vi "Initialize.vi"(8 "error in (no error)":errorcluster) -> (0 "error out":errorcluster, 3 "LiDAR out":refnum<class "Telnet V2.lvclass">)   [LabVIEW 2018]
uses:
  Telnet V2.lvclass
  PPLs/Configuration/Configuration.lvlibp/Configuration.lvclass
  C:/AME Test Engineering/LabVIEW/PPLs/LiDAR/Parent/LiDAR.lvlibp/LiDAR.lvclass
panel:
  in  "PPLs Folder Path":path
  in  "INI File Path":path
  in  "Device":string
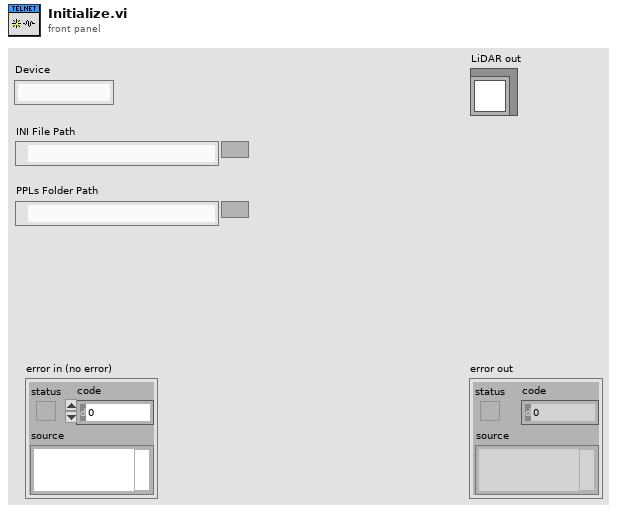
[diagram p1: front panel]
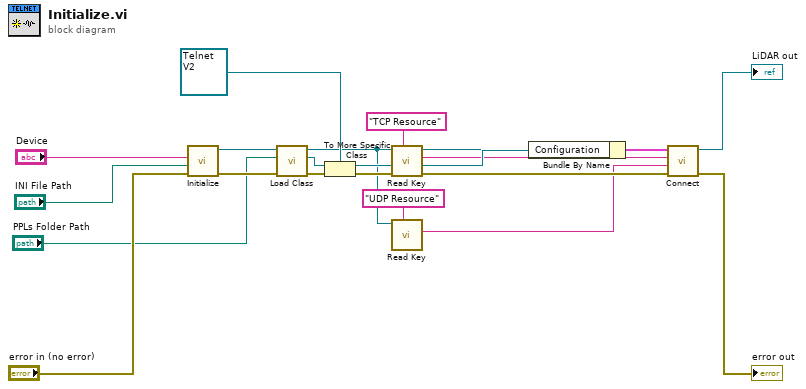
[diagram p0: block diagram]
diagram:
  n1 = call "Initialize.vi"("error in"="error in (no error)", "INI File Path"="INI File Path", "Device"="Device") -> ("error out"=w19:errorcluster, "Configuration out"=w20:refnum<class "Configuration.lvclass">)  [unwired: 7 in]
  n2 = call "Load Class.vi"("error in"=w19, "PPLs Folder Path"="PPLs Folder Path", "Configuration in"=w20) -> ("error out"=w18:errorcluster, "Class out"=w17:refnum<class>, "Configuration out"=w12:refnum<class "Configuration.lvclass">)  [unwired: 6 in]
  n3 = To More Specific Class(target class=refnum<class "Telnet V2.lvclass"> refnum ("LiDAR in"), reference=w17, error in=w18) -> (specific class reference=w14:refnum<class "Telnet V2.lvclass">, error out=w16:errorcluster)
  n4 = call "Read Key.vi"("Key:"="TCP Resource", "error in"=w16, "Configuration in"=w12) -> ("error out"=w5:errorcluster, "Value"=w2:string, "Configuration out"=w10:refnum<class "Configuration.lvclass">)  [unwired: 6 in]
  n5 = call "Read Key.vi"("Key:"="UDP Resource", "Configuration in"=w12) -> ("Value"=w1:string)  [unwired: 7 in, 2 out]
  n6 = Bundle By Name(cluster=w14, "Configuration"=w10) -> (w8:cluster{})
  n7 = call-dynamic "Connect.vi"("error in (no error)"=w5, "UDP Resource"=w1, "TCP Resource"=w2, "Telnet in"=w8) -> ("error out"=→"error out":errorcluster, "Telnet out"=→"LiDAR out":refnum<class "Telnet V2.lvclass">)  [unwired: 6 in]
